vi "1D Wave PDE Solver.vi"(0 "PDE in":refnum<class "NI_PDE.lvclass">, 11 "error in (no error)":errorcluster) -> (4 "PDE out":refnum<class "NI_PDE.lvclass">, 6 "U(t, x)":dbl[][](array[numeric]), 15 "error out":errorcluster)   [LabVIEW 2020, in "NI_PDE.lvlib"]
doc: "Solves a partial differential equation. You must manually select the polymorphic instance to use."
uses:
  <vilib>/gmath/NI_PDE.lvlib
  <vilib>/gmath/pde.llb/PDEClass/NI_PDE.lvclass
  <vilib>/gmath/pde.llb/ICClass/IC_1D_Numeric/NI_IC_1D_Numeric.lvclass
  e:/builds/penguin/labview/branches/2020/dev/dist/vi.lib/gmath/pde.llb/ICClass/NI_IC.lvclass
  <vilib>/gmath/pde.llb/DomainClass/Domain_Evolut_1D/NI_Domain_Evolut_1D.lvclass
  e:/builds/penguin/labview/branches/2020/dev/dist/vi.lib/gmath/pde.llb/DomainClass/NI_Domain.lvclass
  <vilib>/gmath/pde.llb/BCClass/BC_Evolut_1D_Numeric/NI_BC_Evolut_1D_Numeric.lvclass
  e:/builds/penguin/labview/branches/2020/dev/dist/vi.lib/gmath/pde.llb/BCClass/NI_BC.lvclass
  <vilib>/gmath/pde.llb/RHSClass/RHS_2D_Numeric/NI_RHS_2D_Numeric.lvclass
  e:/builds/penguin/labview/branches/2020/dev/dist/vi.lib/gmath/pde.llb/RHSClass/NI_RHS.lvclass
  <vilib>/gmath/pde.llb/PDEClass/PDE_Wave_1D/NI_PDE_Wave_1D.lvclass
  e:/builds/penguin/labview/branches/2020/dev/dist/vi.lib/gmath/pde.llb/PDEClass/NI_PDE.lvclass
  <vilib>/gmath/pde.llb/DomainClass/Domain_Evolut_1D/Domain Data.ctl
  <vilib>/gmath/pde.llb/PDEClass/PDE_2ndOrder_ConstPara/Para Data.ctl
  <vilib>/gmath/pde.llb/PDEClass/PDE Data_Class.ctl
  <vilib>/gmath/pde.llb/RHSClass/NI_RHS.lvclass
  <vilib>/gmath/pde.llb/DomainClass/NI_Domain.lvclass
  <vilib>/gmath/pde.llb/BCClass/NI_BC.lvclass
  <vilib>/gmath/pde.llb/ICClass/NI_IC.lvclass
  <vilib>/gmath/pde.llb/ICClass/IC_1D_Numeric/IC Data.ctl
  <vilib>/gmath/pde.llb/Common/PDE_IC Type.ctl
  <vilib>/gmath/pde.llb/BCClass/BC_Evolut_1D_Numeric/BC Data.ctl
  <vilib>/gmath/pde.llb/Common/PDE_BC Type.ctl
  <vilib>/gmath/pde.llb/Common/PDE_BC Position 1D.ctl
  <vilib>/gmath/pde.llb/PDEClass/PDE_2ndOrder_ConstPara/NI_PDE_2ndOrder_ConstPara.lvclass
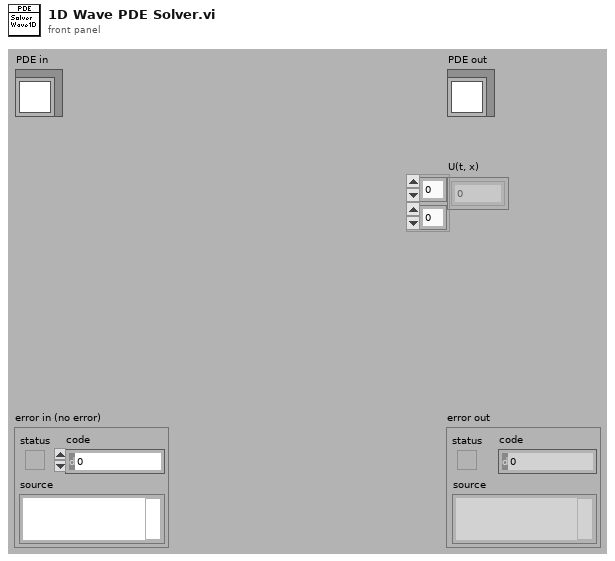
[diagram p1: front panel]
types:
  T1 = typedef "NI_PDE.lvlib/NI_PDE.lvclass/PDE Data_Class.ctl" = cluster{"PDE":refnum<class "NI_PDE.lvclass">, "RHS":refnum<class "NI_RHS.lvclass">, "Domain":refnum<class "NI_Domain.lvclass">, "BC":refnum<class "NI_BC.lvclass">, "IC":refnum<class "NI_IC.lvclass">}
  T2 = typedef "NI_PDE.lvlib/NI_PDE_2ndOrder_ConstPara.lvclass/Para Data.ctl" = cluster{"k":dbl, "a":dbl}
  T3 = typedef "NI_PDE.lvlib/NI_Domain_Evolut_1D.lvclass/Domain Data.ctl" = cluster{"T":cluster{"initial t":dbl, "final t":dbl, "# of t-points":i32}, "X":cluster{"start x":dbl, "end x":dbl, "# of x-points":i32}}
  T4 = typedef "NI_PDE.lvlib/NI_BC_Evolut_1D_Numeric.lvclass/BC Data.ctl" = cluster{"type":T5, "position":T6, "G":dbl[]}
  T5 = typedef "NI_PDE.lvlib/PDE_BC Type.ctl" = i32
  T6 = typedef "NI_PDE.lvlib/PDE_BC Position 1D.ctl" = i32
  T7 = typedef "NI_PDE.lvlib/NI_IC_1D_Numeric.lvclass/IC Data.ctl" = cluster{"type":T8, "H":dbl[]}
  T8 = typedef "NI_PDE.lvlib/PDE_IC Type.ctl" = i32
  T9 = typedef "NI_PDE.lvlib/NI_PDE.lvclass/PDE Data_Variant.ctl" = cluster{"parameter":variant, "RHS":variant, "domain":variant, "BC Array":variant[], "IC Array":variant[]}
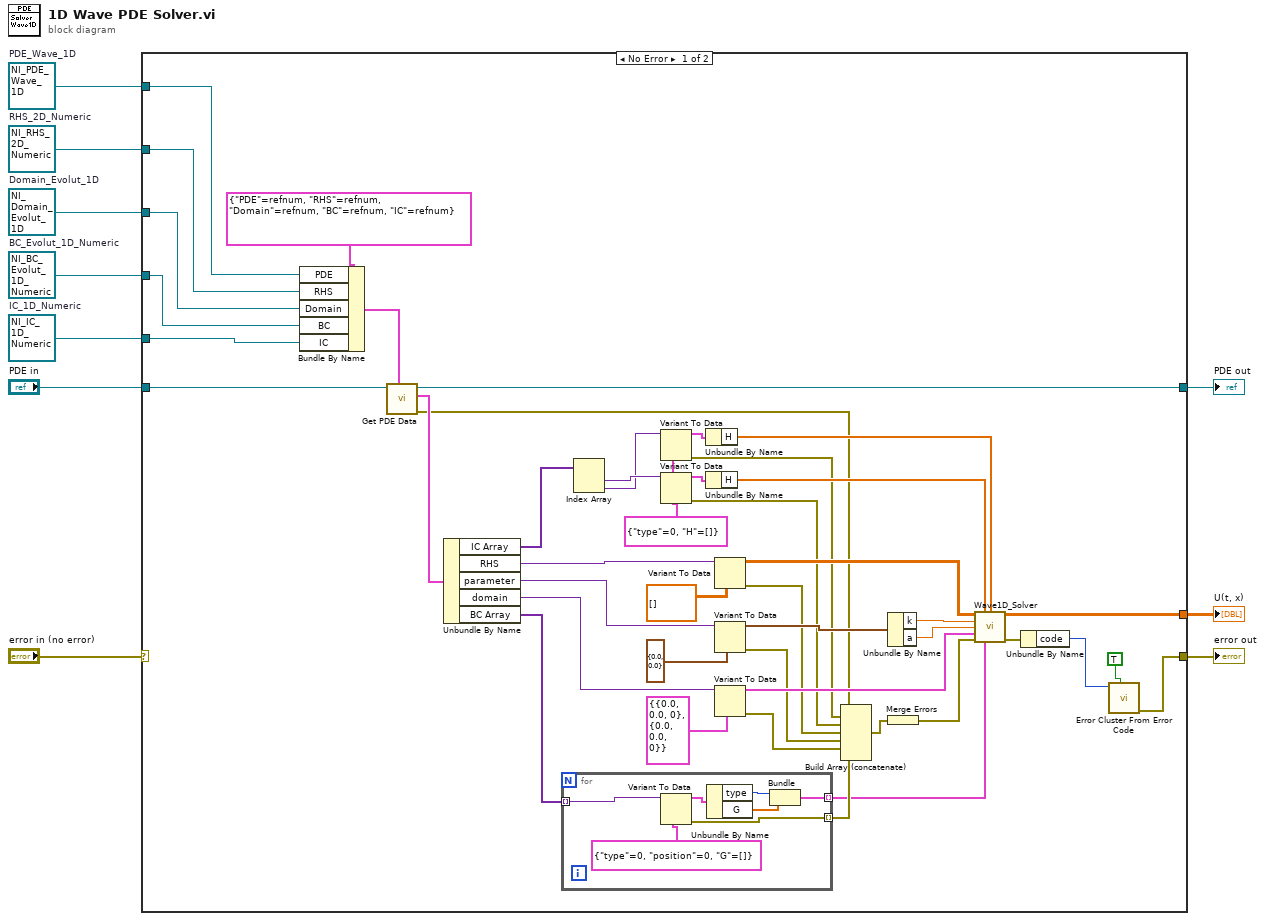
[diagram p0: block diagram]
diagram:
  w6 = refnum<class "NI_PDE_Wave_1D.lvclass"> refnum  # PDE_Wave_1D
  w10 = refnum<class "NI_RHS_2D_Numeric.lvclass"> refnum  # RHS_2D_Numeric
  w8 = refnum<class "NI_BC_Evolut_1D_Numeric.lvclass"> refnum  # BC_Evolut_1D_Numeric
  w9 = refnum<class "NI_Domain_Evolut_1D.lvclass"> refnum  # Domain_Evolut_1D
  w7 = refnum<class "NI_IC_1D_Numeric.lvclass"> refnum  # IC_1D_Numeric
  n1 = case shown="No Error" "error in (no error)" {
    selector: "error in (no error)" -> [_ w63]
    tunnel: [w55 _] -> w2
    tunnel: "PDE in" -> [w35 w64]
    tunnel: [w34 w64] -> w3
    tunnel: [w51 w63] -> w1
    tunnel: w6 -> [w27 _]
    tunnel: w9 -> [w25 _]
    tunnel: w8 -> [w24 _]
    tunnel: w10 -> [w26 _]
    tunnel: w7 -> [w22 _]
    frame No Error {
      w18 = T7 {"type"=0, "H"=[]} ("Initial Value")
      n2 = Bundle By Name(cluster=T1 {"PDE"=refnum, "RHS"=refnum, "Domain"=refnum, "BC"=refnum, "IC"=refnum} ("target class"), "PDE"=w27, "RHS"=w26, "Domain"=w25, "BC"=w24, "IC"=w22) -> (w23:T1)
      n3 = call <vilib>:"Get PDE Data.vi"("target class"=w23, "PDE in"=w35) -> ("error out"=w12:errorcluster, "PDE data"=w33:T9, "PDE out"=w34:refnum<class "NI_PDE.lvclass">)  [unwired: 3 in, 4 out]
      n4 = Unbundle By Name(w33) -> ("IC Array"=w17:variant[], "RHS"=w31:variant, "parameter"=w32:variant, "domain"=w30:variant, "BC Array"=w29:variant[])
      n5 = for {
        tunnel: w29 -> [w61] mode=indexing
        tunnel: [w62] -> w39 mode=indexing
        tunnel: [w57] -> w36 mode=indexing
        n6 = Variant To Data(type=T4 {"type"=0, "position"=0, "G"=[]} ("BC data"), Variant=w61) -> (data=w60:T4, error out=w62:errorcluster)  [unwired: 1 in]
        n7 = Unbundle By Name(w60) -> ("type"=w59:T5, "G"=w58:dbl[])
        n8 = Bundle("type"=w59, "G"=w58) -> (w57:cluster{"type":T5, "G":dbl[]})  [unwired: 1 out]
      }
      n9 = Index Array(array=w17) -> (element #1=w16:variant, element #2=w15:variant)  [unwired: 2 in]
      n10 = Variant To Data(type=w18, Variant=w15) -> (data=w19:T7, error out=w11:errorcluster)  [unwired: 1 in]
      n11 = Variant To Data(type=w18, Variant=w16) -> (data=w20:T7, error out=w21:errorcluster)  [unwired: 1 in]
      n12 = Unbundle By Name(w19) -> ("H"=w13:dbl[])
      n13 = Unbundle By Name(w20) -> ("H"=w14:dbl[])
      n14 = Variant To Data(type=dbl[][] [] ("F(x, y)"), Variant=w31) -> (data=w43:dbl[][], error out=w42:errorcluster)  [unwired: 1 in]
      n15 = Variant To Data(type=T2 {"k"=0.0, "a"=0.0} ("para data"), Variant=w32) -> (data=w47:T2, error out=w41:errorcluster)  [unwired: 1 in]
      n16 = Variant To Data(type=T3 {"T"={"initial t"=0.0, "final t"=0.0, "# of t-points"=0}, "X"={"start x"=0.0, "end x"=0.0, "# of x-points"=0}} ("domain data"), Variant=w30) -> (data=w49:T3, error out=w40:errorcluster)  [unwired: 1 in]
      n17 = Build Array (concatenate)(w12, w11, w21, w42, w41, w40, w39) -> (w38:errorcluster[])
      n18 = Unbundle By Name(w47) -> ("k"=w46:dbl, "a"=w45:dbl)
      n19 = Merge Errors(w38) -> (w37:errorcluster)
      n20 = call <vilib>:"Wave1D_Solver.vi"("F(t, x)"=w43, "Initial Value"=w14, "Initial Derivative"=w13, "k"=w46, "a"=w45, "Domain"=w49, "error in (no error)"=w37, "Boundary Condition"=w36) -> ("U(t, x)"=w55:dbl[][], "error out"=w52:errorcluster)  [unwired: 6 out]
      n21 = Unbundle By Name(w52) -> ("code"=w54:i32)
      n22 = call <vilib>:"Error Cluster From Error Code.vi"("show call chain? (False)"=TRUE, "error code (0)"=w54) -> ("error out"=w51:errorcluster)  [unwired: 1 in, 6 out]
    }
    frame Error {
    }
  }
  "U(t, x)" <- w2
  "error out" <- w1
  "PDE out" <- w3
